vi "sub vi - Read Analog All v9.11.vi"() -> (2 "Analog loop time":dbl, 3 "array GRAPH":dynamicdata[](array[waveform]), 4 "LAB01":T2, 6 "LAB02":T3, 8 "LAB03":T4, 10 "LAB04":T5, 13 "deg C":dbl, 14 "Any Error":bool, 15 "LAB05":T6)   [LabVIEW 2013]
uses:
  program files/Global display 3.vi
  <vilib>/measure/mascope.llb/Amplitude and Levels 1 chan.vi
  <vilib>/addons/Electrical Power/Basic/Measurement/Power (1 Channel).vi
  <vilib>/addons/Electrical Power/Basic/Measurement/RMS (N Channels).vi
  <vilib>/addons/Electrical Power/Basic/Measurement/RMS (1 Channel).vi
  <vilib>/addons/Electrical Power/Basic/NI_EP_Basic.lvlib
  <vilib>/measure/NI_MAPro.lvlib
panel:
  in  "Tab Control":T1(tab)
  out "LAB01-2 (PF)":dbl
  out "LAB01-1 (PF)":dbl
  out "LAB01-2 (V)":dbl
  out "LAB01-2 (A)":dbl
  out "LAB01-1 (V)":dbl
  out "LAB01-1 (A)":dbl
  out "LAB01-2 (GRAPH)":dynamicdata(graph)
  out "LAB01-1 (GRAPH)":dynamicdata(graph)
  out "LAB02-2 (PF)":dbl
  out "LAB02-1 (PF)":dbl
  out "LAB02-2 (V)":dbl
  out "LAB02-2 (A)":dbl
  out "LAB02-1 (V)":dbl
  out "LAB02-1 (A)":dbl
  out "LAB02-2 (GRAPH)":dynamicdata(graph)
  out "LAB02-1 (GRAPH)":dynamicdata(graph)
  out "LAB03-2 (PF)":dbl
  out "LAB03-1 (PF)":dbl
  out "LAB03-2 (V)":dbl
  out "LAB03-2 (A)":dbl
  out "LAB03-1 (V)":dbl
  out "LAB03-1 (A)":dbl
  out "LAB03-2 (GRAPH)":dynamicdata(graph)
  out "LAB03-1 (GRAPH)":dynamicdata(graph)
  out "LAB04-2 (PF)":dbl
  out "LAB04-1 (PF)":dbl
  out "LAB04-2 (V)":dbl
  out "LAB04-2 (A)":dbl
  out "LAB04-1 (V)":dbl
  out "LAB04-1 (A)":dbl
  out "LAB04-1 (GRAPH)":dynamicdata(graph)
  out "LAB04-2 (GRAPH)":dynamicdata(graph)
  out "LAB05-2 (PF)":dbl
  out "LAB05-1 (PF)":dbl
  out "LAB05-2 (V)":dbl
  out "LAB05-2 (A)":dbl
  out "LAB05-1 (V)":dbl
  out "LAB05-1 (A)":dbl
  out "LAB05-1 (GRAPH)":dynamicdata(graph)
  out "LAB05-2 (GRAPH)":dynamicdata(graph)
  out "A1 error":errorcluster
  out "array ERROR":errorcluster[](array[cluster])
  out "AI2-OFF":dynamicdata(graph)
  out "AI2-ON":dynamicdata(graph)
  out "AI1-OFF":dynamicdata(graph)
  out "AI1-ON":dynamicdata(graph)
  out "AI0-OFF":dynamicdata(graph)
  out "AI0-ON":dynamicdata(graph)
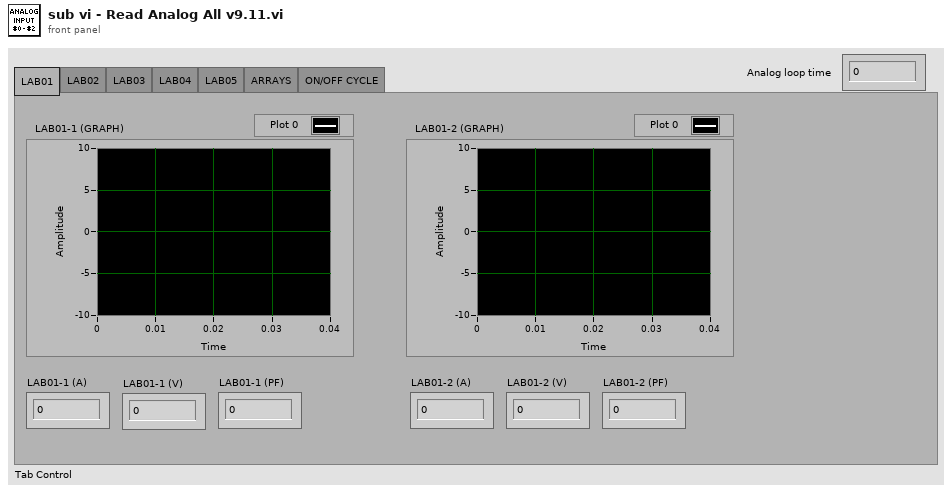
[diagram p1: front panel]
types:
  T1 = enum32{"LAB01", "LAB02", "LAB03", "LAB04", "LAB05", "ARRAYS", "ON/OFF CYCLE"}
  T2 = cluster{"LAB01-1 (A)":dbl, "LAB01-1 (V)":dbl, "LAB01-1 (PF)":dbl, "LAB01-2 (A)":dbl, "LAB01-2 (V)":dbl, "LAB01-2 (PF)":dbl}
  T3 = cluster{"LAB02-1 (A)":dbl, "LAB02-1 (V)":dbl, "LAB02-1 (PF)":dbl, "LAB02-2 (A)":dbl, "LAB02-2 (V)":dbl, "LAB02-2 (PF)":dbl}
  T4 = cluster{"LAB03-1 (A)":dbl, "LAB03-1 (V)":dbl, "LAB03-1 (PF)":dbl, "LAB03-2 (A)":dbl, "LAB03-2 (V)":dbl, "LAB03-2 (PF)":dbl}
  T5 = cluster{"LAB04-1 (A)":dbl, "LAB04-1 (V)":dbl, "LAB04-1 (PF)":dbl, "LAB04-2 (A)":dbl, "LAB04-2 (V)":dbl, "LAB04-2 (PF)":dbl}
  T6 = cluster{"LAB05-1 (A)":dbl, "LAB05-1 (V)":dbl, "LAB05-1 (PF)":dbl, "LAB05-2 (A)":dbl, "LAB05-2 (V)":dbl, "LAB05-2 (PF)":dbl}
  T7 = typedef "NI_EP_Basic.lvlib/basic_Power Value.ctl" = cluster{"active power [W]":dbl, "apparent power [VA]":dbl, "reactive power [VAR]":dbl, "power factor":dbl}
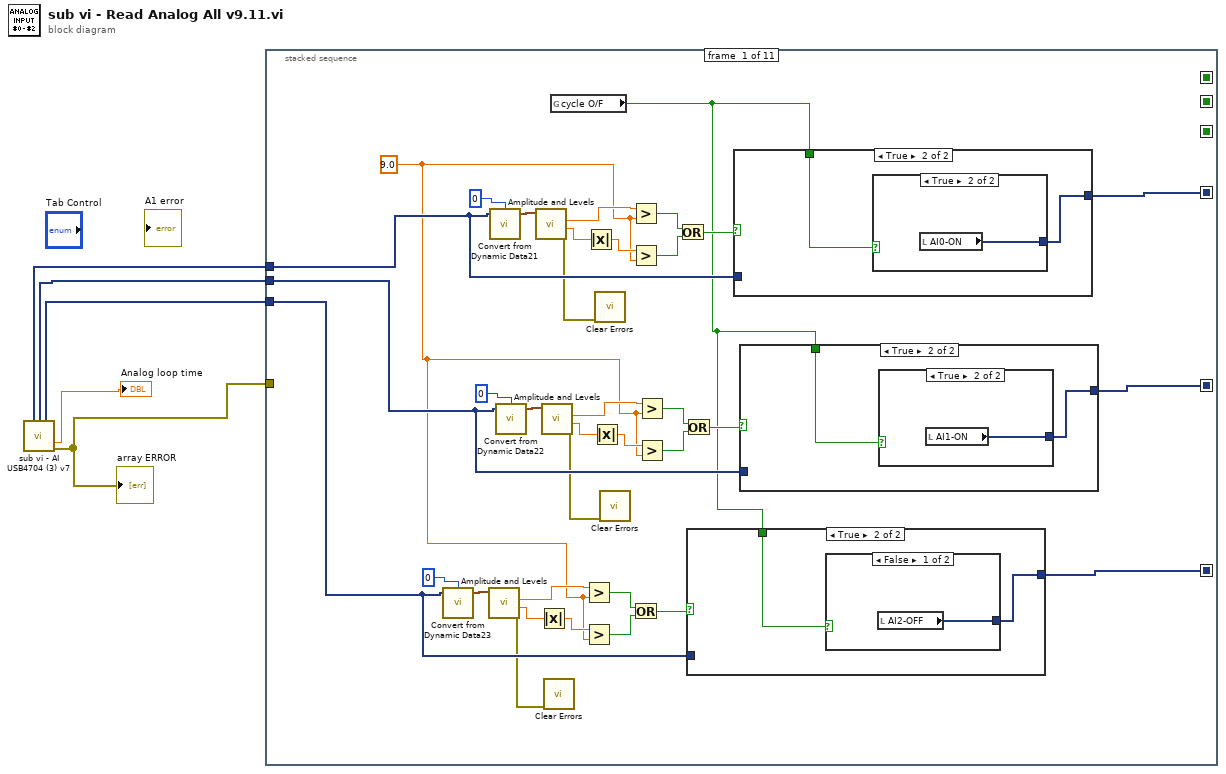
[diagram p0: block diagram]
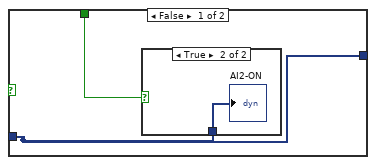
[diagram p2: hidden frame]
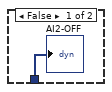
[diagram p3: hidden frame]
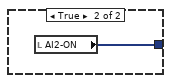
[diagram p4: hidden frame]
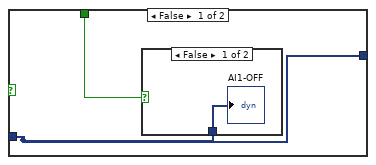
[diagram p5: hidden frame]
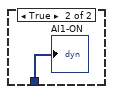
[diagram p6: hidden frame]
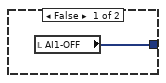
[diagram p7: hidden frame]
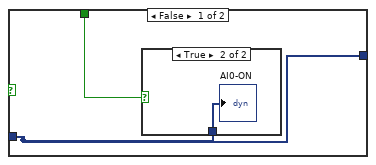
[diagram p8: hidden frame]
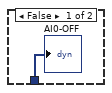
[diagram p9: hidden frame]
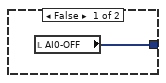
[diagram p10: hidden frame]
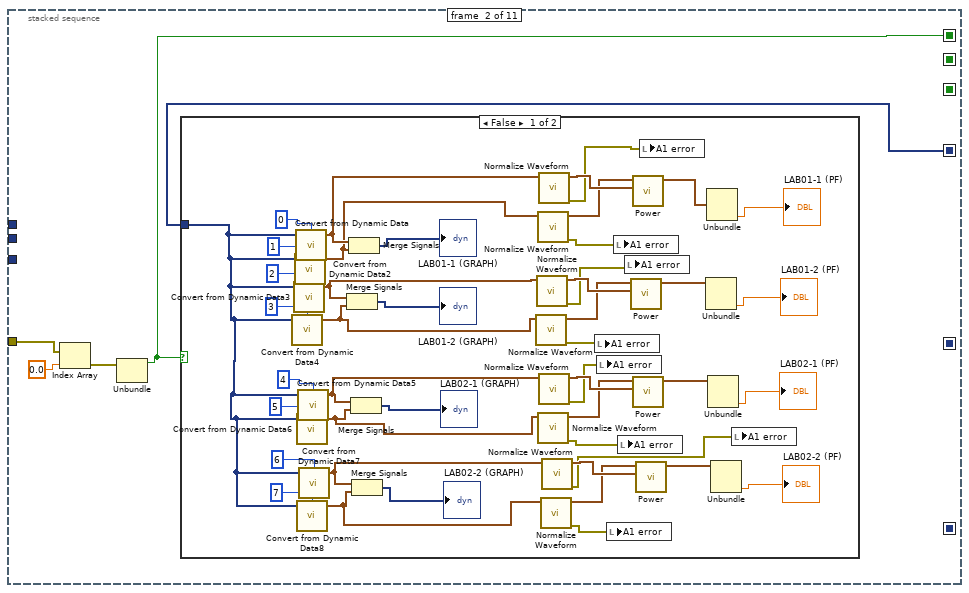
[diagram p11: hidden frame]
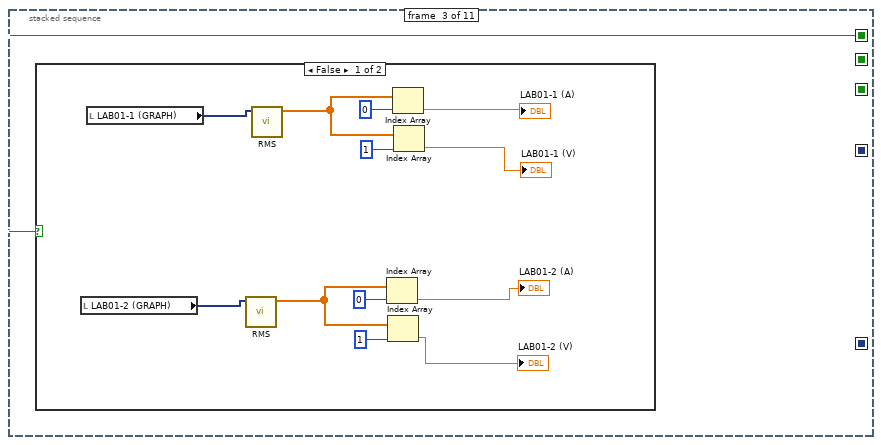
[diagram p13: hidden frame]
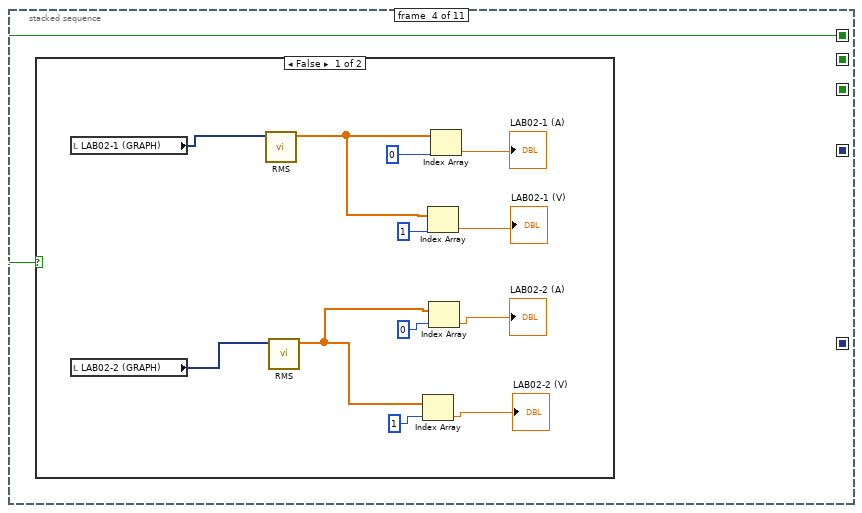
[diagram p15: hidden frame]
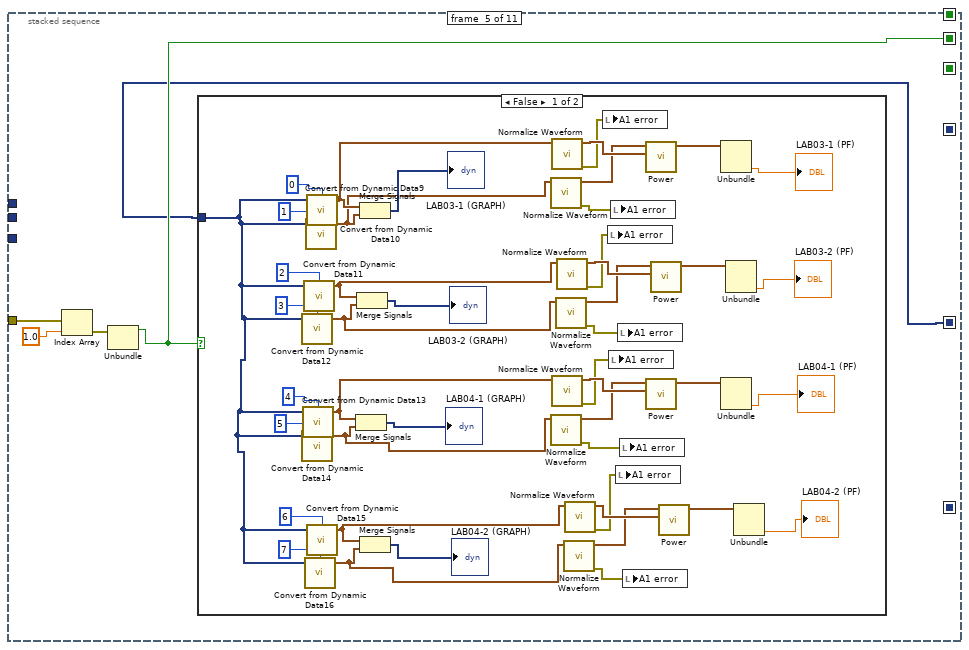
[diagram p17: hidden frame]
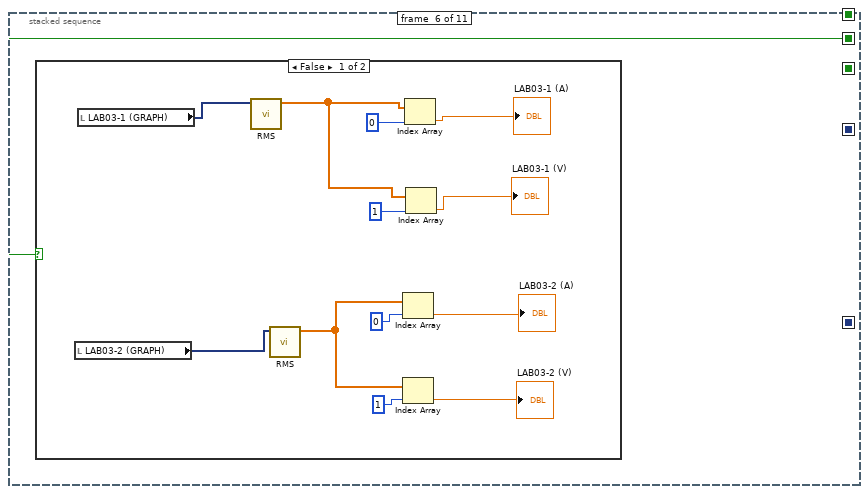
[diagram p19: hidden frame]
diagram:
  n1 = call "sub vi - AI USB4704 (3) v7.vi"() -> ("Graph 1"=w5:dynamicdata, "Graph 2"=w4:dynamicdata, "Graph 3"=w3:dynamicdata, "loop time"=→"Analog loop time":dbl, "error array"=w1:errorcluster[])  [unwired: 11 in]
  "array ERROR" <- w1
  n2 = stacked-sequence {
    seq-local: [_ w66 _ _ _ _ _ _ _ _ _] -> [_ _ w115 w128 _ _ _ _ _ _ w275]
    seq-local: [_ _ _ _ w142 _ _ _ _ _ _] -> [_ _ _ _ _ w191 w204 _ _ _ w274]
    seq-local: [_ _ _ _ _ _ _ w218 _ _ _] -> [_ _ _ _ _ _ _ _ w248 _ w273]
    seq-local: [w32 _ _ _ _ _ _ _ _ _ _] -> [_ w65 _ _ _ _ _ _ _ _ _]
    seq-local: [w21 _ _ _ _ _ _ _ _ _ _] -> [_ _ _ _ w141 _ _ _ _ _ _]
    seq-local: [w9 _ _ _ _ _ _ _ _ _ _] -> [_ _ _ _ _ _ _ w217 _ _ _]
    tunnel: w5 -> [w31 _ _ _ _ _ _ _ _ _ _]
    tunnel: w4 -> [w22 _ _ _ _ _ _ _ _ _ _]
    tunnel: w3 -> [w12 _ _ _ _ _ _ _ _ _ _]
    tunnel: w1 -> [_ w69 _ _ w145 _ _ w221 _ _ _]
    frame #0 {
      w11 = 9.0
      n3 = call "Convert from Dynamic Data23"("Dynamic Data Type"=w12, "Channel"=0) -> ("Waveform"=w19:waveform(dbl))  [unwired: 2 in]
      n4 = call-poly <vilib>:"Amplitude and Levels.vi"("signal in"=w19) -> ("error out"=w6:errorcluster, "low state level"=w18:dbl, "high state level"=w17:dbl)  [unwired: 7 in, 1 out]
      n5 = call "Convert from Dynamic Data21"("Dynamic Data Type"=w31, "Channel"=0) -> ("Waveform"=w39:waveform(dbl))  [unwired: 2 in]
      n6 = call "Convert from Dynamic Data22"("Dynamic Data Type"=w22, "Channel"=0) -> ("Waveform"=w29:waveform(dbl))  [unwired: 2 in]
      n7 = call-poly <vilib>:"Amplitude and Levels.vi"("signal in"=w39) -> ("error out"=w8:errorcluster, "low state level"=w38:dbl, "high state level"=w37:dbl)  [unwired: 7 in, 1 out]
      n8 = Absolute Value(x=w18) -> (abs(x)=w16:dbl)
      n9 = call-poly <vilib>:"Amplitude and Levels.vi"("signal in"=w29) -> ("error out"=w7:errorcluster, "low state level"=w28:dbl, "high state level"=w27:dbl)  [unwired: 7 in, 1 out]
      n10 = call <vilib>:"Clear Errors.vi"("error in (no error)"=w6) -> ()  [unwired: 6 in, 1 out]
      n11 = global read "Global display 3.vi" "cycle O/F"() -> (w10:bool)
      n12 = Greater?(x=w17, y=w11) -> (0:w15:bool)
      n13 = Greater?(x=w16, y=w11) -> (0:w14:bool)
      n14 = Absolute Value(x=w38) -> (abs(x)=w36:dbl)
      n15 = Absolute Value(x=w28) -> (abs(x)=w26:dbl)
      n16 = call <vilib>:"Clear Errors.vi"("error in (no error)"=w8) -> ()  [unwired: 6 in, 1 out]
      n17 = call <vilib>:"Clear Errors.vi"("error in (no error)"=w7) -> ()  [unwired: 6 in, 1 out]
      n18 = Greater?(x=w37, y=w11) -> (0:w35:bool)
      n19 = Greater?(x=w36, y=w11) -> (0:w34:bool)
      n20 = Or(x=w15, y=w14) -> (x .or. y?=w13:bool)
      n21 = Greater?(x=w27, y=w11) -> (0:w25:bool)
      n22 = Greater?(x=w26, y=w11) -> (0:w24:bool)
      n23 = Or(x=w35, y=w34) -> (x .or. y?=w33:bool)
      n24 = Or(x=w25, y=w24) -> (x .or. y?=w23:bool)
      n25 = case shown="True" w13 {
        tunnel: w10 -> [w42 w46]
        tunnel: [w41 w45] -> w9
        tunnel: w12 -> [w41 _]
        frame False {
          n26 = case shown="True" w42 {
            tunnel: w41 -> [w43 w44]
            frame False {
              "AI2-OFF" <- w43
            }
            frame True {
              "AI2-ON" <- w44
            }
          }
        }
        frame True {
          n27 = case shown="False" w46 {
            tunnel: [w47 w48] -> w45
            frame False {
              n28 = local read "AI2-OFF"() -> (w47:dynamicdata)
            }
            frame True {
              n29 = local read "AI2-ON"() -> (w48:dynamicdata)
            }
          }
        }
      }
      n30 = case shown="True" w33 {
        tunnel: w10 -> [w58 w62]
        tunnel: [w57 w61] -> w32
        tunnel: w31 -> [w57 _]
        frame False {
          n31 = case shown="True" w58 {
            tunnel: w57 -> [w59 w60]
            frame False {
              "AI0-OFF" <- w59
            }
            frame True {
              "AI0-ON" <- w60
            }
          }
        }
        frame True {
          n32 = case shown="True" w62 {
            tunnel: [w63 w64] -> w61
            frame False {
              n33 = local read "AI0-OFF"() -> (w63:dynamicdata)
            }
            frame True {
              n34 = local read "AI0-ON"() -> (w64:dynamicdata)
            }
          }
        }
      }
      n35 = case shown="True" w23 {
        tunnel: w10 -> [w50 w54]
        tunnel: [w49 w53] -> w21
        tunnel: w22 -> [w49 _]
        frame False {
          n36 = case shown="False" w50 {
            tunnel: w49 -> [w51 w52]
            frame False {
              "AI1-OFF" <- w51
            }
            frame True {
              "AI1-ON" <- w52
            }
          }
        }
        frame True {
          n37 = case shown="True" w54 {
            tunnel: [w55 w56] -> w53
            frame False {
              n38 = local read "AI1-OFF"() -> (w55:dynamicdata)
            }
            frame True {
              n39 = local read "AI1-ON"() -> (w56:dynamicdata)
            }
          }
        }
      }
    }
    frame #1 {
      n40 = Index Array(array=w69, index=0.0) -> (element=w67:errorcluster)
      n41 = Unbundle(w67) -> ("status"=w66:bool)  [unwired: 2 out]
      n42 = case shown="False" w66 {
        tunnel: w65 -> [w104 _]
        frame False {
          n43 = call "Convert from Dynamic Data4"("Dynamic Data Type"=w104, "Channel"=3) -> ("Waveform"=w90:waveform(dbl))  [unwired: 2 in]
          n44 = call "Convert from Dynamic Data3"("Dynamic Data Type"=w104, "Channel"=2) -> ("Waveform"=w91:waveform(dbl))  [unwired: 2 in]
          n45 = call "Convert from Dynamic Data2"("Dynamic Data Type"=w104, "Channel"=1) -> ("Waveform"=w100:waveform(dbl))  [unwired: 2 in]
          n46 = call "Convert from Dynamic Data"("Dynamic Data Type"=w104, "Channel"=0) -> ("Waveform"=w101:waveform(dbl))  [unwired: 2 in]
          n47 = call "Convert from Dynamic Data6"("Dynamic Data Type"=w104, "Channel"=5) -> ("Waveform"=w85:waveform(dbl))  [unwired: 2 in]
          n48 = call "Convert from Dynamic Data8"("Dynamic Data Type"=w104, "Channel"=7) -> ("Waveform"=w79:waveform(dbl))  [unwired: 2 in]
          n49 = call "Convert from Dynamic Data5"("Dynamic Data Type"=w104, "Channel"=4) -> ("Waveform"=w86:waveform(dbl))  [unwired: 2 in]
          n50 = call "Convert from Dynamic Data7"("Dynamic Data Type"=w104, "Channel"=6) -> ("Waveform"=w80:waveform(dbl))  [unwired: 2 in]
          n51 = Merge Signals(w91, w90) -> (→"LAB01-2 (GRAPH)":dynamicdata)
          n52 = Merge Signals(w101, w100) -> (→"LAB01-1 (GRAPH)":dynamicdata)
          n53 = Merge Signals(w86, w85) -> (→"LAB02-1 (GRAPH)":dynamicdata)
          n54 = Merge Signals(w80, w79) -> (→"LAB02-2 (GRAPH)":dynamicdata)
          n55 = call <vilib>:"Normalize Waveform.vi"("waveform in"=w90) -> ("error out"=w74:errorcluster, "normalized waveform"=w94:waveform(dbl))  [unwired: 7 in, 2 out]
          n56 = call <vilib>:"Normalize Waveform.vi"("waveform in"=w91) -> ("error out"=w75:errorcluster, "normalized waveform"=w95:waveform(dbl))  [unwired: 7 in, 2 out]
          n57 = call <vilib>:"Normalize Waveform.vi"("waveform in"=w100) -> ("error out"=w76:errorcluster, "normalized waveform"=w98:waveform(dbl))  [unwired: 7 in, 2 out]
          n58 = call <vilib>:"Normalize Waveform.vi"("waveform in"=w85) -> ("error out"=w72:errorcluster, "normalized waveform"=w88:waveform(dbl))  [unwired: 7 in, 2 out]
          n59 = call <vilib>:"Normalize Waveform.vi"("waveform in"=w101) -> ("error out"=w77:errorcluster, "normalized waveform"=w99:waveform(dbl))  [unwired: 7 in, 2 out]
          n60 = call <vilib>:"Normalize Waveform.vi"("waveform in"=w86) -> ("error out"=w73:errorcluster, "normalized waveform"=w89:waveform(dbl))  [unwired: 7 in, 2 out]
          n61 = call <vilib>:"Normalize Waveform.vi"("waveform in"=w79) -> ("error out"=w70:errorcluster, "normalized waveform"=w82:waveform(dbl))  [unwired: 7 in, 2 out]
          n62 = call <vilib>:"Normalize Waveform.vi"("waveform in"=w80) -> ("error out"=w71:errorcluster, "normalized waveform"=w83:waveform(dbl))  [unwired: 7 in, 2 out]
          n63 = local write "A1 error"(w74) -> ()
          n64 = local write "A1 error"(w73) -> ()
          n65 = local write "A1 error"(w70) -> ()
          n66 = local write "A1 error"(w76) -> ()
          n67 = local write "A1 error"(w72) -> ()
          n68 = local write "A1 error"(w75) -> ()
          n69 = call-poly <vilib>:"Power.vi"("current waveform"=w95, "voltage waveform"=w94) -> ("power value"=w93:T7)  [unwired: 8 in, 1 out]
          n70 = call-poly <vilib>:"Power.vi"("current waveform"=w99, "voltage waveform"=w98) -> ("power value"=w97:T7)  [unwired: 8 in, 1 out]
          n71 = call-poly <vilib>:"Power.vi"("current waveform"=w89, "voltage waveform"=w88) -> ("power value"=w87:T7)  [unwired: 8 in, 1 out]
          n72 = call-poly <vilib>:"Power.vi"("current waveform"=w83, "voltage waveform"=w82) -> ("power value"=w81:T7)  [unwired: 8 in, 1 out]
          n73 = local write "A1 error"(w77) -> ()
          n74 = Unbundle(w93) -> ("power factor"=→"LAB01-2 (PF)":dbl)  [unwired: 3 out]
          n75 = Unbundle(w97) -> ("power factor"=→"LAB01-1 (PF)":dbl)  [unwired: 3 out]
          n76 = Unbundle(w87) -> ("power factor"=→"LAB02-1 (PF)":dbl)  [unwired: 3 out]
          n77 = Unbundle(w81) -> ("power factor"=→"LAB02-2 (PF)":dbl)  [unwired: 3 out]
          n78 = local write "A1 error"(w71) -> ()
        }
        frame True {
        }
      }
    }
    frame #2 {
      n79 = case shown="False" w115 {
        frame False {
          n80 = local read "LAB01-2 (GRAPH)"() -> (w124:dynamicdata)
          n81 = local read "LAB01-1 (GRAPH)"() -> (w118:dynamicdata)
          n82 = call-poly <vilib>:"RMS.vi"("waveforms"=w124) -> ("RMS values"=w123:dbl[])  [unwired: 9 in, 1 out]
          n83 = call-poly <vilib>:"RMS.vi"("waveforms"=w118) -> ("RMS values"=w127:dbl[])  [unwired: 9 in, 1 out]
          n84 = Index Array(array=w123, index=0) -> (element=→"LAB01-2 (A)":dbl)
          n85 = Index Array(array=w123, index=1) -> (element=→"LAB01-2 (V)":dbl)
          n86 = Index Array(array=w127, index=0) -> (element=→"LAB01-1 (A)":dbl)
          n87 = Index Array(array=w127, index=1) -> (element=→"LAB01-1 (V)":dbl)
        }
        frame True {
        }
      }
    }
    frame #3 {
      n88 = case shown="False" w128 {
        frame False {
          n89 = local read "LAB02-1 (GRAPH)"() -> (w136:dynamicdata)
          n90 = local read "LAB02-2 (GRAPH)"() -> (w132:dynamicdata)
          n91 = call-poly <vilib>:"RMS.vi"("waveforms"=w136) -> ("RMS values"=w135:dbl[])  [unwired: 9 in, 1 out]
          n92 = call-poly <vilib>:"RMS.vi"("waveforms"=w132) -> ("RMS values"=w131:dbl[])  [unwired: 9 in, 1 out]
          n93 = Index Array(array=w131, index=1) -> (element=→"LAB02-2 (V)":dbl)
          n94 = Index Array(array=w135, index=1) -> (element=→"LAB02-1 (V)":dbl)
          n95 = Index Array(array=w131, index=0) -> (element=→"LAB02-2 (A)":dbl)
          n96 = Index Array(array=w135, index=0) -> (element=→"LAB02-1 (A)":dbl)
        }
        frame True {
        }
      }
    }
    frame #4 {
      n97 = Index Array(array=w145, index=1.0) -> (element=w143:errorcluster)
      n98 = Unbundle(w143) -> ("status"=w142:bool)  [unwired: 2 out]
      n99 = case shown="False" w142 {
        tunnel: w141 -> [w178 _]
        frame False {
          n100 = call "Convert from Dynamic Data12"("Dynamic Data Type"=w178, "Channel"=3) -> ("Waveform"=w167:waveform(dbl))  [unwired: 2 in]
          n101 = call "Convert from Dynamic Data14"("Dynamic Data Type"=w178, "Channel"=5) -> ("Waveform"=w161:waveform(dbl))  [unwired: 2 in]
          n102 = call "Convert from Dynamic Data13"("Dynamic Data Type"=w178, "Channel"=4) -> ("Waveform"=w162:waveform(dbl))  [unwired: 2 in]
          n103 = call "Convert from Dynamic Data11"("Dynamic Data Type"=w178, "Channel"=2) -> ("Waveform"=w168:waveform(dbl))  [unwired: 2 in]
          n104 = call "Convert from Dynamic Data16"("Dynamic Data Type"=w178, "Channel"=7) -> ("Waveform"=w155:waveform(dbl))  [unwired: 2 in]
          n105 = call "Convert from Dynamic Data10"("Dynamic Data Type"=w178, "Channel"=1) -> ("Waveform"=w173:waveform(dbl))  [unwired: 2 in]
          n106 = call "Convert from Dynamic Data9"("Dynamic Data Type"=w178, "Channel"=0) -> ("Waveform"=w174:waveform(dbl))  [unwired: 2 in]
          n107 = call "Convert from Dynamic Data15"("Dynamic Data Type"=w178, "Channel"=6) -> ("Waveform"=w156:waveform(dbl))  [unwired: 2 in]
          n108 = Merge Signals(w162, w161) -> (→"LAB04-1 (GRAPH)":dynamicdata)
          n109 = Merge Signals(w168, w167) -> (→"LAB03-2 (GRAPH)":dynamicdata)
          n110 = Merge Signals(w174, w173) -> (→"LAB03-1 (GRAPH)":dynamicdata)
          n111 = Merge Signals(w156, w155) -> (→"LAB04-2 (GRAPH)":dynamicdata)
          n112 = call <vilib>:"Normalize Waveform.vi"("waveform in"=w173) -> ("error out"=w152:errorcluster, "normalized waveform"=w176:waveform(dbl))  [unwired: 7 in, 2 out]
          n113 = call <vilib>:"Normalize Waveform.vi"("waveform in"=w161) -> ("error out"=w148:errorcluster, "normalized waveform"=w164:waveform(dbl))  [unwired: 7 in, 2 out]
          n114 = call <vilib>:"Normalize Waveform.vi"("waveform in"=w174) -> ("error out"=w153:errorcluster, "normalized waveform"=w177:waveform(dbl))  [unwired: 7 in, 2 out]
          n115 = call <vilib>:"Normalize Waveform.vi"("waveform in"=w162) -> ("error out"=w149:errorcluster, "normalized waveform"=w165:waveform(dbl))  [unwired: 7 in, 2 out]
          n116 = call <vilib>:"Normalize Waveform.vi"("waveform in"=w167) -> ("error out"=w150:errorcluster, "normalized waveform"=w170:waveform(dbl))  [unwired: 7 in, 2 out]
          n117 = call <vilib>:"Normalize Waveform.vi"("waveform in"=w168) -> ("error out"=w151:errorcluster, "normalized waveform"=w171:waveform(dbl))  [unwired: 7 in, 2 out]
          n118 = call <vilib>:"Normalize Waveform.vi"("waveform in"=w155) -> ("error out"=w146:errorcluster, "normalized waveform"=w158:waveform(dbl))  [unwired: 7 in, 2 out]
          n119 = call <vilib>:"Normalize Waveform.vi"("waveform in"=w156) -> ("error out"=w147:errorcluster, "normalized waveform"=w159:waveform(dbl))  [unwired: 7 in, 2 out]
          n120 = local write "A1 error"(w153) -> ()
          n121 = local write "A1 error"(w151) -> ()
          n122 = local write "A1 error"(w149) -> ()
          n123 = local write "A1 error"(w152) -> ()
          n124 = local write "A1 error"(w147) -> ()
          n125 = local write "A1 error"(w150) -> ()
          n126 = local write "A1 error"(w148) -> ()
          n127 = local write "A1 error"(w146) -> ()
          n128 = call-poly <vilib>:"Power.vi"("current waveform"=w177, "voltage waveform"=w176) -> ("power value"=w175:T7)  [unwired: 8 in, 1 out]
          n129 = call-poly <vilib>:"Power.vi"("current waveform"=w165, "voltage waveform"=w164) -> ("power value"=w163:T7)  [unwired: 8 in, 1 out]
          n130 = call-poly <vilib>:"Power.vi"("current waveform"=w171, "voltage waveform"=w170) -> ("power value"=w169:T7)  [unwired: 8 in, 1 out]
          n131 = call-poly <vilib>:"Power.vi"("current waveform"=w159, "voltage waveform"=w158) -> ("power value"=w157:T7)  [unwired: 8 in, 1 out]
          n132 = Unbundle(w175) -> ("power factor"=→"LAB03-1 (PF)":dbl)  [unwired: 3 out]
          n133 = Unbundle(w163) -> ("power factor"=→"LAB04-1 (PF)":dbl)  [unwired: 3 out]
          n134 = Unbundle(w169) -> ("power factor"=→"LAB03-2 (PF)":dbl)  [unwired: 3 out]
          n135 = Unbundle(w157) -> ("power factor"=→"LAB04-2 (PF)":dbl)  [unwired: 3 out]
        }
        frame True {
        }
      }
    }
    frame #5 {
      n136 = case shown="False" w191 {
        frame False {
          n137 = local read "LAB03-2 (GRAPH)"() -> (w198:dynamicdata)
          n138 = local read "LAB03-1 (GRAPH)"() -> (w199:dynamicdata)
          n139 = call-poly <vilib>:"RMS.vi"("waveforms"=w199) -> ("RMS values"=w197:dbl[])  [unwired: 9 in, 1 out]
          n140 = call-poly <vilib>:"RMS.vi"("waveforms"=w198) -> ("RMS values"=w194:dbl[])  [unwired: 9 in, 1 out]
          n141 = Index Array(array=w194, index=0) -> (element=→"LAB03-2 (A)":dbl)
          n142 = Index Array(array=w194, index=1) -> (element=→"LAB03-2 (V)":dbl)
          n143 = Index Array(array=w197, index=0) -> (element=→"LAB03-1 (A)":dbl)
          n144 = Index Array(array=w197, index=1) -> (element=→"LAB03-1 (V)":dbl)
        }
        frame True {
        }
      }
    }
    frame #6 {
      n145 = case shown="False" w204 {
        frame False {
          n146 = local read "LAB04-1 (GRAPH)"() -> (w212:dynamicdata)
          n147 = local read "LAB04-2 (GRAPH)"() -> (w208:dynamicdata)
          n148 = call-poly <vilib>:"RMS.vi"("waveforms"=w212) -> ("RMS values"=w211:dbl[])  [unwired: 9 in, 1 out]
          n149 = call-poly <vilib>:"RMS.vi"("waveforms"=w208) -> ("RMS values"=w207:dbl[])  [unwired: 9 in, 1 out]
          n150 = Index Array(array=w207, index=0) -> (element=→"LAB04-2 (A)":dbl)
          n151 = Index Array(array=w211, index=0) -> (element=→"LAB04-1 (A)":dbl)
          n152 = Index Array(array=w207, index=1) -> (element=→"LAB04-2 (V)":dbl)
          n153 = Index Array(array=w211, index=1) -> (element=→"LAB04-1 (V)":dbl)
        }
        frame True {
        }
      }
    }
    frame #7 {
      n154 = Index Array(array=w221, index=2.0) -> (element=w219:errorcluster)
      n155 = Unbundle(w219) -> ("status"=w218:bool)  [unwired: 2 out]
      n156 = case shown="False" w218 {
        tunnel: w217 -> [w224 _]
        frame False {
          n157 = call "Convert from Dynamic Data18"("Dynamic Data Type"=w224, "Channel"=1) -> ("Waveform"=w237:waveform(dbl))  [unwired: 2 in]
          n158 = call "Convert from Dynamic Data20"("Dynamic Data Type"=w224, "Channel"=3) -> ("Waveform"=w231:waveform(dbl))  [unwired: 2 in]
          n159 = call "Convert from Dynamic Data17"("Dynamic Data Type"=w224, "Channel"=0) -> ("Waveform"=w238:waveform(dbl))  [unwired: 2 in]
          n160 = call "Convert from Dynamic Data19"("Dynamic Data Type"=w224, "Channel"=2) -> ("Waveform"=w232:waveform(dbl))  [unwired: 2 in]
          n161 = Merge Signals(w238, w237) -> (→"LAB05-1 (GRAPH)":dynamicdata)
          n162 = Merge Signals(w232, w231) -> (→"LAB05-2 (GRAPH)":dynamicdata)
          n163 = call "Convert from Dynamic Data24"("Dynamic Data Type"=w224, "Channel"=4) -> ("Waveform"=w223:waveform(dbl))  [unwired: 2 in]
          n164 = call-poly <vilib>:"RMS.vi"("waveform"=w223) -> ("RMS value"=→"deg C":dbl)  [unwired: 9 in, 1 out]
          n165 = call <vilib>:"Normalize Waveform.vi"("waveform in"=w237) -> ("error out"=w229:errorcluster, "normalized waveform"=w240:waveform(dbl))  [unwired: 7 in, 2 out]
          n166 = call <vilib>:"Normalize Waveform.vi"("waveform in"=w238) -> ("error out"=w228:errorcluster, "normalized waveform"=w241:waveform(dbl))  [unwired: 7 in, 2 out]
          n167 = call <vilib>:"Normalize Waveform.vi"("waveform in"=w231) -> ("error out"=w227:errorcluster, "normalized waveform"=w234:waveform(dbl))  [unwired: 7 in, 2 out]
          n168 = call <vilib>:"Normalize Waveform.vi"("waveform in"=w232) -> ("error out"=w226:errorcluster, "normalized waveform"=w235:waveform(dbl))  [unwired: 7 in, 2 out]
          n169 = local write "A1 error"(w227) -> ()
          n170 = local write "A1 error"(w228) -> ()
          n171 = local write "A1 error"(w226) -> ()
          n172 = call-poly <vilib>:"Power.vi"("current waveform"=w241, "voltage waveform"=w240) -> ("power value"=w239:T7)  [unwired: 8 in, 1 out]
          n173 = local write "A1 error"(w229) -> ()
          n174 = call-poly <vilib>:"Power.vi"("current waveform"=w235, "voltage waveform"=w234) -> ("power value"=w233:T7)  [unwired: 8 in, 1 out]
          n175 = Unbundle(w239) -> ("power factor"=→"LAB05-1 (PF)":dbl)  [unwired: 3 out]
          n176 = Unbundle(w233) -> ("power factor"=→"LAB05-2 (PF)":dbl)  [unwired: 3 out]
        }
        frame True {
        }
      }
    }
    frame #8 {
      n177 = case shown="False" w248 {
        frame False {
          n178 = local read "LAB05-2 (GRAPH)"() -> (w255:dynamicdata)
          n179 = local read "LAB05-1 (GRAPH)"() -> (w256:dynamicdata)
          n180 = call-poly <vilib>:"RMS.vi"("waveforms"=w256) -> ("RMS values"=w254:dbl[])  [unwired: 9 in, 1 out]
          n181 = call-poly <vilib>:"RMS.vi"("waveforms"=w255) -> ("RMS values"=w253:dbl[])  [unwired: 9 in, 1 out]
          n182 = Index Array(array=w254, index=1) -> (element=→"LAB05-1 (V)":dbl)
          n183 = Index Array(array=w254, index=0) -> (element=→"LAB05-1 (A)":dbl)
          n184 = Index Array(array=w253, index=1) -> (element=→"LAB05-2 (V)":dbl)
          n185 = Index Array(array=w253, index=0) -> (element=→"LAB05-2 (A)":dbl)
        }
        frame True {
        }
      }
    }
    frame #9 {
      n186 = local read "LAB05-1 (GRAPH)"() -> (w263:dynamicdata)
      n187 = local read "LAB05-2 (GRAPH)"() -> (w262:dynamicdata)
      n188 = local read "LAB04-2 (GRAPH)"() -> (w264:dynamicdata)
      n189 = local read "LAB02-2 (GRAPH)"() -> (w268:dynamicdata)
      n190 = local read "LAB03-1 (GRAPH)"() -> (w267:dynamicdata)
      n191 = local read "LAB04-1 (GRAPH)"() -> (w265:dynamicdata)
      n192 = local read "LAB03-2 (GRAPH)"() -> (w266:dynamicdata)
      n193 = local read "LAB02-1 (GRAPH)"() -> (w269:dynamicdata)
      n194 = local read "LAB01-2 (GRAPH)"() -> (w270:dynamicdata)
      n195 = local read "LAB01-1 (GRAPH)"() -> (w271:dynamicdata)
      n196 = Build Array(w271, w270, w269, w268, w267, w266, w265, w264, w263, w262) -> (→"array GRAPH":dynamicdata[])
    }
    frame #10 {
      n197 = case shown="False" w274 {
        frame False {
          n198 = local read "LAB03-2 (PF)"() -> (w292:dbl)
          n199 = local read "LAB03-1 (PF)"() -> (w295:dbl)
          n200 = local read "LAB03-1 (A)"() -> (w297:dbl)
          n201 = local read "LAB03-1 (V)"() -> (w296:dbl)
          n202 = local read "LAB03-2 (A)"() -> (w294:dbl)
          n203 = local read "LAB03-2 (V)"() -> (w293:dbl)
          n204 = Bundle("LAB03-1 (A)"=w297, "LAB03-1 (V)"=w296, "LAB03-1 (PF)"=w295, "LAB03-2 (A)"=w294, "LAB03-2 (V)"=w293, "LAB03-2 (PF)"=w292) -> (→"LAB03":T4)  [unwired: 1 in]
          n205 = local read "LAB04-1 (PF)"() -> (w289:dbl)
          n206 = local read "LAB04-2 (PF)"() -> (w286:dbl)
          n207 = local read "LAB04-1 (A)"() -> (w291:dbl)
          n208 = local read "LAB04-1 (V)"() -> (w290:dbl)
          n209 = local read "LAB04-2 (A)"() -> (w288:dbl)
          n210 = local read "LAB04-2 (V)"() -> (w287:dbl)
          n211 = Bundle("LAB04-1 (A)"=w291, "LAB04-1 (V)"=w290, "LAB04-1 (PF)"=w289, "LAB04-2 (A)"=w288, "LAB04-2 (V)"=w287, "LAB04-2 (PF)"=w286) -> (→"LAB04":T5)  [unwired: 1 in]
        }
        frame True {
        }
      }
      n212 = case shown="False" w275 {
        frame False {
          n213 = local read "LAB01-1 (PF)"() -> (w302:dbl)
          n214 = local read "LAB01-2 (PF)"() -> (w299:dbl)
          n215 = local read "LAB01-1 (V)"() -> (w303:dbl)
          n216 = local read "LAB01-2 (A)"() -> (w301:dbl)
          n217 = local read "LAB01-2 (V)"() -> (w300:dbl)
          n218 = local read "LAB01-1 (A)"() -> (w304:dbl)
          n219 = Bundle("LAB01-1 (A)"=w304, "LAB01-1 (V)"=w303, "LAB01-1 (PF)"=w302, "LAB01-2 (A)"=w301, "LAB01-2 (V)"=w300, "LAB01-2 (PF)"=w299) -> (→"LAB01":T2)  [unwired: 1 in]
          n220 = local read "LAB02-2 (PF)"() -> (w306:dbl)
          n221 = local read "LAB02-1 (PF)"() -> (w309:dbl)
          n222 = local read "LAB02-2 (A)"() -> (w308:dbl)
          n223 = local read "LAB02-2 (V)"() -> (w307:dbl)
          n224 = local read "LAB02-1 (V)"() -> (w310:dbl)
          n225 = local read "LAB02-1 (A)"() -> (w311:dbl)
          n226 = Bundle("LAB02-1 (A)"=w311, "LAB02-1 (V)"=w310, "LAB02-1 (PF)"=w309, "LAB02-2 (A)"=w308, "LAB02-2 (V)"=w307, "LAB02-2 (PF)"=w306) -> (→"LAB02":T3)  [unwired: 1 in]
        }
        frame True {
        }
      }
      n227 = case shown="False" w273 {
        frame False {
          n228 = local read "LAB05-2 (PF)"() -> (w278:dbl)
          n229 = local read "LAB05-1 (PF)"() -> (w281:dbl)
          n230 = local read "LAB05-2 (V)"() -> (w279:dbl)
          n231 = local read "LAB05-1 (A)"() -> (w283:dbl)
          n232 = local read "LAB05-1 (V)"() -> (w282:dbl)
          n233 = local read "LAB05-2 (A)"() -> (w280:dbl)
          n234 = Bundle("LAB05-1 (A)"=w283, "LAB05-1 (V)"=w282, "LAB05-1 (PF)"=w281, "LAB05-2 (A)"=w280, "LAB05-2 (V)"=w279, "LAB05-2 (PF)"=w278) -> (→"LAB05":T6)  [unwired: 1 in]
        }
        frame True {
        }
      }
      n235 = Or(x=w275, y=w274) -> (x .or. y?=w276:bool)
      n236 = Or(x=w276, y=w273) -> (x .or. y?=→"Any Error":bool)
    }
  }
